vi "홍미4.vi"() -> ()   [LabVIEW 2015]
uses:
  <vilib>/NXT/Block Support/NXT_InputPort.ctl
  <vilib>/NXT/Block Support/NXT_OutputPort.ctl
  <vilib>/NXT/Dual Mode Library/Sensors/Sonar_cm.vi
  <vilib>/NXT/NXTIO Xnodes/NXTIONodeSubVIs/NXTMoveMotors.vi
  <vilib>/NXT/Dual Mode Library/Sensors/Light_On.vi
  <vilib>/NXT/NXTIO Xnodes/NXTIONodeSubVIs/LEGOStopAllMotors.vi
  <vilib>/NXT/Dual Mode Library/Waits/Wait_Num.vi
  <vilib>/NXT/Subs/LVHSConnector.ctl
  <vilib>/NXT/NXTIO Xnodes/AddressXNode/NXTIOAddress.xnode
  <vilib>/NXT/NXTIO Xnodes/NXTIOXNode/NXTIO.xnode
  <vilib>/NXT/LegoClasses/BrickReference/BrickReference.lvclass
panel:
  in  "stop":bool
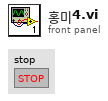
[diagram p1: front panel]
types:
  T1 = typedef "NXT_OutputPort.ctl" = u8
  T2 = typedef "NXT_InputPort.ctl" = u32
  T3 = typedef "LVHSConnector.ctl" = refnum<class "BrickReference.lvclass">
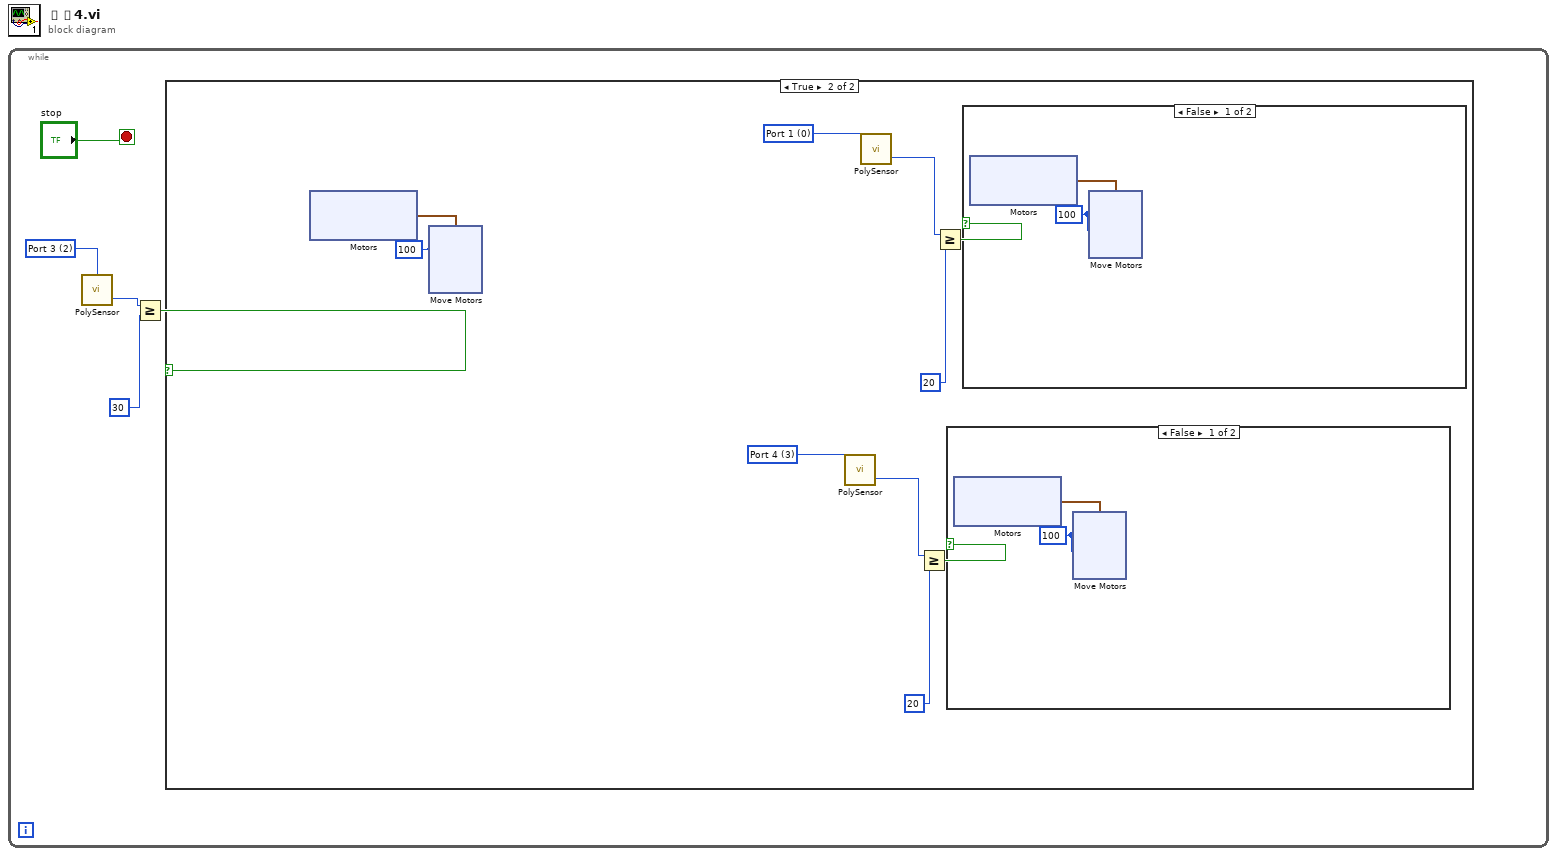
[diagram p0: block diagram]
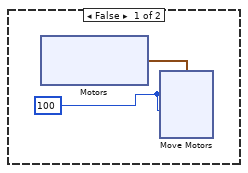
[diagram p2: hidden frame]
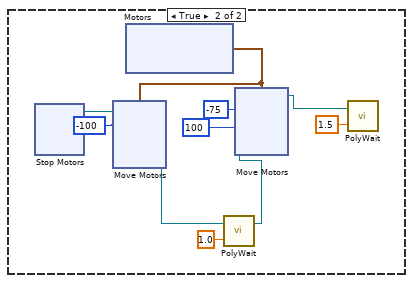
[diagram p3: hidden frame]
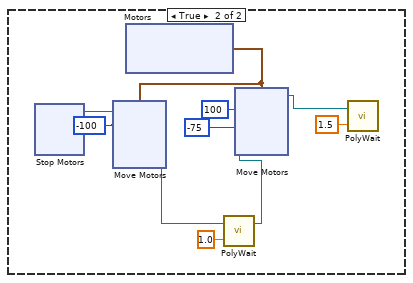
[diagram p4: hidden frame]
diagram:
  n1 = while {
    stop <- "stop" stop-if-true
    w5 = T2 2 items=["Port 1", "Port 2", "Port 3", "Port 4"] ("Port (Port 4)")
    n2 = call-poly <vilib>:"PolySensor.vi"("Port (Port 4)"=w5) -> ("Distance (cm)"=w4:i16)  [unwired: 2 in, 1 out]
    n3 = Greater Or Equal?(x=w4, y=i16 30) -> (x >= y?=w2:bool)
    n4 = case shown="True" w2 {
      frame False {
        w6 = i8 100 ("Power/Speed 1")
        n5 = xnode "Motors"() -> ("Motor"=w7:cluster{"Port":T1, "Port":T1})
        n6 = xnode "Move Motors"("Power/Speed 2"=w6, "Power/Speed 1"=w6, "Motors"=w7) -> ()  [unwired: 1 in, 1 out]
      }
      frame True {
        w17 = T2 3 items=["Port 1", "Port 2", "Port 3", "Port 4"] ("Port (Port 3)")
        w21 = i8 100 ("Power/Speed 1")
        w23 = T2 0 items=["Port 1", "Port 2", "Port 3", "Port 4"] ("Port (Port 3)")
        n7 = xnode "Motors"() -> ("Motor"=w22:cluster{"Port":T1, "Port":T1})
        n8 = xnode "Move Motors"("Power/Speed 1"=w21, "Motors"=w22, "Power/Speed 2"=w21) -> ()  [unwired: 1 in, 1 out]
        n9 = call-poly <vilib>:"PolySensor.vi"("Port (Port 3)"=w17) -> ("Scaled Value"=w19:i16)  [unwired: 2 in, 1 out]
        n10 = call-poly <vilib>:"PolySensor.vi"("Port (Port 3)"=w23) -> ("Scaled Value"=w25:i16)  [unwired: 2 in, 1 out]
        n11 = Greater Or Equal?(x=w19, y=i16 20) -> (x >= y?=w20:bool)
        n12 = Greater Or Equal?(x=w25, y=i16 20) -> (x >= y?=w26:bool)
        n13 = case shown="False" w20 {
          frame False {
            w27 = i8 100 ("Power/Speed 1")
            n14 = xnode "Motors"() -> ("Motor"=w28:cluster{"Port":T1, "Port":T1})
            n15 = xnode "Move Motors"("Power/Speed 2"=w27, "Power/Speed 1"=w27, "Motors"=w28) -> ()  [unwired: 1 in, 1 out]
          }
          frame True {
            w42 = i8 -100 ("Power/Speed 1")
            n16 = xnode "Stop Motors"() -> ("NXT/EV3"=w38:T3)  [unwired: 2 in]
            n17 = xnode "Motors"() -> ("Motor"=w43:cluster{"Port":T1, "Port":T1})
            n18 = xnode "Move Motors"("Power/Speed 2"=w42, "Power/Speed 1"=w42, "Motors"=w43, "NXT/EV3"=w38) -> ("NXT/EV3"=w41:T3)
            n19 = call-poly <vilib>:"PolyWait.vi"("Time (1 sec)"=sgl 1.0, "NXT/EV3"=w41) -> ("NXT/EV3"=w40:T3)  [unwired: 2 in]
            n20 = xnode "Move Motors"("Power/Speed 2"=i8 100, "Power/Speed 1"=i8 -75, "Motors"=w43, "NXT/EV3"=w40) -> ("NXT/EV3"=w47:T3)
            n21 = call-poly <vilib>:"PolyWait.vi"("Time (1 sec)"=sgl 1.5, "NXT/EV3"=w47) -> ()  [unwired: 2 in, 1 out]
          }
        }
        n22 = case shown="False" w26 {
          frame False {
            w77 = i8 100 ("Power/Speed 1")
            n23 = xnode "Motors"() -> ("Motor"=w78:cluster{"Port":T1, "Port":T1})
            n24 = xnode "Move Motors"("Power/Speed 2"=w77, "Power/Speed 1"=w77, "Motors"=w78) -> ()  [unwired: 1 in, 1 out]
          }
          frame True {
            w92 = i8 -100 ("Power/Speed 1")
            n25 = xnode "Stop Motors"() -> ("NXT/EV3"=w88:T3)  [unwired: 2 in]
            n26 = xnode "Motors"() -> ("Motor"=w93:cluster{"Port":T1, "Port":T1})
            n27 = xnode "Move Motors"("Power/Speed 2"=w92, "Power/Speed 1"=w92, "Motors"=w93, "NXT/EV3"=w88) -> ("NXT/EV3"=w91:T3)
            n28 = call-poly <vilib>:"PolyWait.vi"("Time (1 sec)"=sgl 1.0, "NXT/EV3"=w91) -> ("NXT/EV3"=w90:T3)  [unwired: 2 in]
            n29 = xnode "Move Motors"("Power/Speed 2"=i8 -75, "Power/Speed 1"=i8 100, "Motors"=w93, "NXT/EV3"=w90) -> ("NXT/EV3"=w97:T3)
            n30 = call-poly <vilib>:"PolyWait.vi"("Time (1 sec)"=sgl 1.5, "NXT/EV3"=w97) -> ()  [unwired: 2 in, 1 out]
          }
        }
      }
    }
  }
